vi "Tool File Paths.vi"(11 "error in (no error)":errorcluster) -> (4 "Tool Configuration File Path":path, 6 "Database File Paths":T1, 15 "error out":errorcluster)   [LabVIEW 2023, in "Utilities.lvlib"]
uses:
  Utilities.lvlib
  Hotel Management Tool Model/Hotel Management Tool Model/Database File Paths.ctl
  Hotel Management Tool Model/Hotel Management Tool Model/Hotel Management Tool Model.lvclass
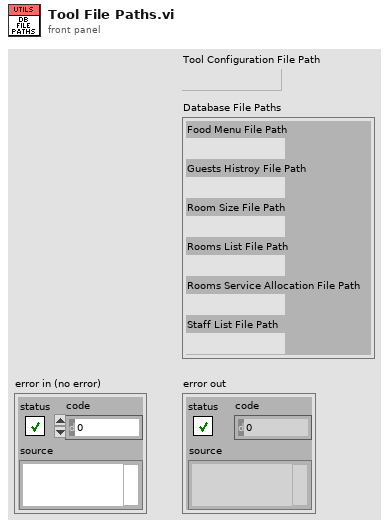
[diagram p1: front panel]
types:
  T1 = typedef "Hotel Management Tool Model.lvlib/Hotel Management Tool Model.lvclass/Database File Paths.ctl" = cluster{"Food Menu File Path":path, "Guests Histroy File Path":path, "Room Size File Path":path, "Rooms List File Path":path, "Rooms Service Allocation File Path":path, "Staff List File Path":path}
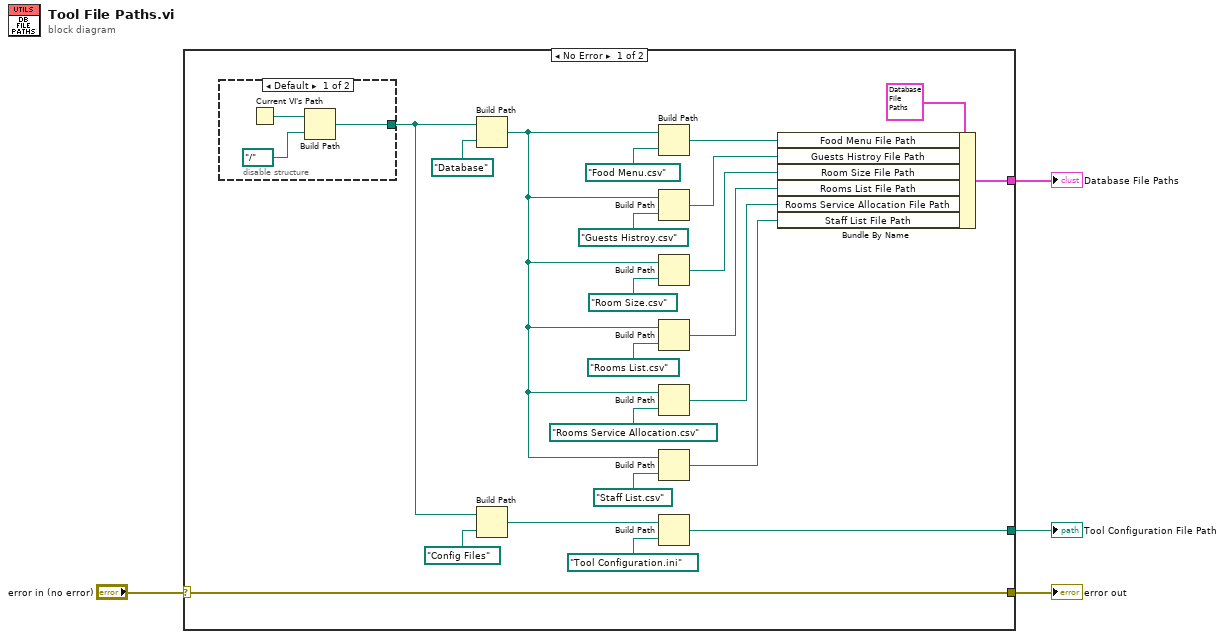
[diagram p0: block diagram]
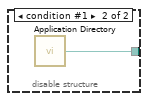
[diagram p2: hidden frame]
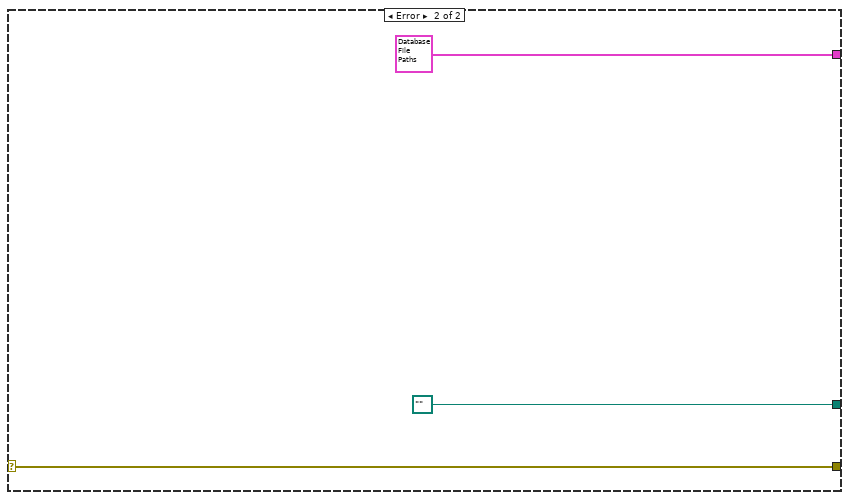
[diagram p3: hidden frame]
diagram:
  n1 = case shown="No Error" "error in (no error)" {
    selector: "error in (no error)" -> [w5 w33]
    tunnel: [w14 path "" ("appended path")] -> w4
    tunnel: [w6 T1 {"Food Menu File Path"=path "", "Guests Histroy File Path"=path "", "Room Size File Path"=path "", "Rooms List File Path"=path "", "Rooms Service Allocation File Path"=path "", "Staff List File Path"=path ""} ("Database File Paths")] -> w3
    tunnel: [w5 w33] -> w1
    frame No Error {
      n2 = disable-structure shown="Default" {
        disable-tunnel: [w27 w30] -> w24
        frame condition #0 (active) {
          n3 = Current VI's Path() -> (path=w29:path)
          n4 = Build Path(base path=w29, name or relative path=path "../.." ("Path")) -> (appended path=w27:path)
        }
        frame condition #1 {
          n5 = call <vilib>:"Application Directory.vi"() -> ("Application Directory"=w30:path)
        }
      }
      n6 = Build Path(base path=w24, name or relative path=path "Database" ("Path")) -> (appended path=w15:path)
      n7 = Build Path(base path=w24, name or relative path=path "Config Files" ("Path")) -> (appended path=w23:path)
      n8 = Build Path(base path=w15, name or relative path=path "Food Menu.csv" ("Path")) -> (appended path=w12:path)
      n9 = Build Path(base path=w15, name or relative path=path "Guests Histroy.csv" ("Path")) -> (appended path=w7:path)
      n10 = Build Path(base path=w15, name or relative path=path "Room Size.csv" ("Path 2")) -> (appended path=w8:path)
      n11 = Build Path(base path=w15, name or relative path=path "Rooms List.csv" ("Path 3")) -> (appended path=w9:path)
      n12 = Build Path(base path=w15, name or relative path=path "Rooms Service Allocation.csv" ("Path 4")) -> (appended path=w10:path)
      n13 = Build Path(base path=w15, name or relative path=path "Staff List.csv" ("Path 5")) -> (appended path=w11:path)
      n14 = Build Path(base path=w23, name or relative path=path "Tool Configuration.ini" ("Path")) -> (appended path=w14:path)
      n15 = Bundle By Name(cluster=T1 {"Food Menu File Path"=path "", "Guests Histroy File Path"=path "", "Room Size File Path"=path "", "Rooms List File Path"=path "", "Rooms Service Allocation File Path"=path "", "Staff List File Path"=path ""} ("Database File Paths"), "Food Menu File Path"=w12, "Guests Histroy File Path"=w7, "Room Size File Path"=w8, "Rooms List File Path"=w9, "Rooms Service Allocation File Path"=w10, "Staff List File Path"=w11) -> (w6:T1)
    }
    frame Error {
    }
  }
  "error out" <- w1
  "Tool Configuration File Path" <- w4
  "Database File Paths" <- w3
